vi "Extract_Province_List.vi"(11 "Country Data In":string[][](array[string])) -> (0 "Province List":string[](array[string]), 3 "Country Data Out":string[][](array[string]))   [LabVIEW 2015]
doc: "This VI extracts the province or states from the csv file to populate the drop-down menu. A lot of these rows of data were deprecated from the file by JHU/CSSE on March 21, 2020"
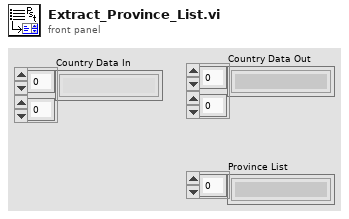
[diagram p1: front panel]
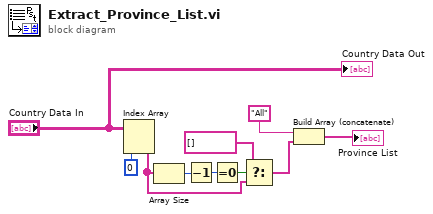
[diagram p0: block diagram]
diagram:
  n1 = Index Array(array="Country Data In", index (col)=0 ("index (row)")) -> (element=w10:string[])  [unwired: 1 in]
  n2 = Array Size(array=w10) -> (size(s)=w4:i32)
  n3 = Decrement(x=w4) -> (x-1=w5:i32)
  n4 = Equal To 0?(x=w5) -> (x = 0?=w6:bool)
  n5 = Select(t=string[] [], s=w6, f=w10) -> (s? t:f=w7:string[])
  n6 = Build Array (concatenate)("All", w7) -> (→"Province List":string[])
  "Country Data Out" <- "Country Data In"
